vi "All sensors.vi"(0 "VISA resource name":refnum<visa-resource-name>, 5 "error in (no error)":errorcluster) -> (6 "Sample Insert (A)":dbl format="%.4f", 8 "Sample Tube (B)":dbl format="%.4f", 10 "1.5K Pot (C)":dbl format="%.4f", 12 "Cold Head (D)":dbl format="%.4f", 14 "VISA resource name out":refnum<visa-resource-name>, 19 "error out":errorcluster)   [LabVIEW 2024]
uses:
  <instrlib>/Lake Shore 336/Public/Data/Sensor Data (Single Reading).vi
  <instrlib>/Lake Shore 336/Lake Shore 336.lvlib
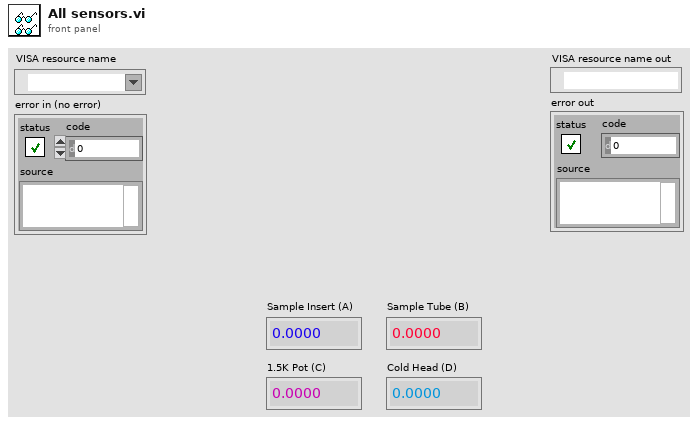
[diagram p1: front panel]
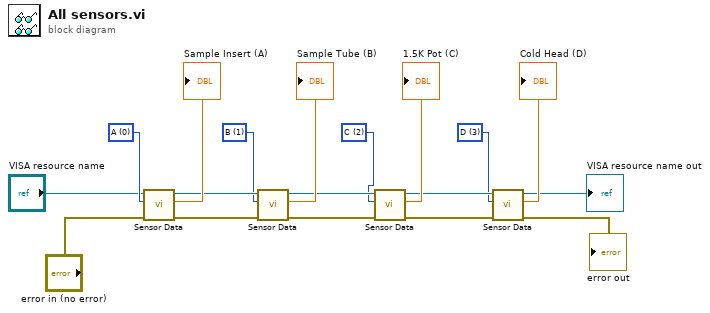
[diagram p0: block diagram]
diagram:
  w7 = u16 3 items=["A", "B", "C", "D"] ("Input (0:A)")
  w6 = u16 2 items=["A", "B", "C", "D"] ("Input (0:A)")
  w8 = u16 1 items=["A", "B", "C", "D"] ("Input (0:A)")
  w5 = u16 0 items=["A", "B", "C", "D"] ("Input (0:A)")
  n1 = call-poly <instrlib>:"Sensor Data.vi"("error in (no error)"="error in (no error)", "Input (0:A)"=w5, "VISA resource name"="VISA resource name") -> ("error out"=w12:errorcluster, "Sensor Data"=→"Sample Insert (A)":dbl, "VISA resource name out"=w9:refnum<visa-resource-name>)  [unwired: 6 in]
  n2 = call-poly <instrlib>:"Sensor Data.vi"("error in (no error)"=w12, "Input (0:A)"=w8, "VISA resource name"=w9) -> ("error out"=w13:errorcluster, "Sensor Data"=→"Sample Tube (B)":dbl, "VISA resource name out"=w10:refnum<visa-resource-name>)  [unwired: 6 in]
  n3 = call-poly <instrlib>:"Sensor Data.vi"("error in (no error)"=w13, "Input (0:A)"=w6, "VISA resource name"=w10) -> ("error out"=w14:errorcluster, "Sensor Data"=→"1.5K Pot (C)":dbl, "VISA resource name out"=w11:refnum<visa-resource-name>)  [unwired: 6 in]
  n4 = call-poly <instrlib>:"Sensor Data.vi"("error in (no error)"=w14, "Input (0:A)"=w7, "VISA resource name"=w11) -> ("error out"=→"error out":errorcluster, "Sensor Data"=→"Cold Head (D)":dbl, "VISA resource name out"=→"VISA resource name out":refnum<visa-resource-name>)  [unwired: 6 in]
